vi "Event structure.vi"() -> ()   [LabVIEW 2021]
panel:
  in  "stop":bool
  in  "OK Button":bool
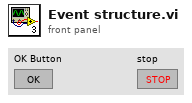
[diagram p1: front panel]
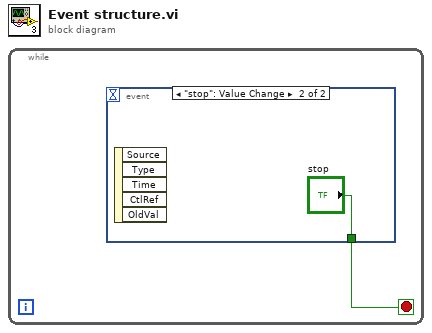
[diagram p0: block diagram]
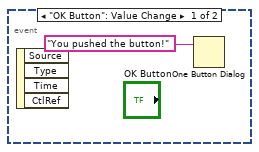
[diagram p2: hidden frame]
diagram:
  n1 = while {
    stop <- w1 stop-if-true
    n2 = event shown="[1] \"stop\": Value Change" {
      selector: _ -> [_ _]
      dyn-events: _ -> [_ _]
      timeout: _ -> [_ _]
      tunnel: [_ "stop"] -> w1
      event "OK Button": Value Change {
        n3 = event-data() -> ()  [unwired: 1 in, 4 out]
        n4 = One Button Dialog(message="You pushed the button!") -> ()  [unwired: 1 in, 1 out]
      }
      event "stop": Value Change {
        n5 = event-data() -> ()  [unwired: 1 in, 5 out]
      }
    }
  }
